vi "PID.vi"(9 "setpoint":dbl[](array[numeric])=[0.0] caption="设定值" format="%.2f", 10 "Relay":bool, 11 "Custom FPGA Reference Out":refnum<k20>) -> ()   [LabVIEW 2017, in "年前程序.lvlib"]
uses:
  <vilib>/Utility/error.llb/Error Cluster From Error Code.vi
  <vilib>/rvi/errors/niLvFpgaAdjustHostInterfaceError.vi
  <vilib>/addons/control/pid/pid.llb/PID (DBL Array).vi
  <vilib>/rvi/interface/nirviReadWriteControl/nirviReadWriteControl.xnode
  <vilib>/addons/control/pid/NI_PID_pid.lvlib
  NiFpgaLv.dll
  <vilib>/rvi/interface/Simulation/niFpgaSimulationCallBeginRW.vi
panel:
  in  "PID gains":T1={"proportional gain (Kc)"=0.0001, "integral time (Ti, min)"=3e-06, "derivative time (Td, min)"=0.0} {"proportional gain (Kc)" format="%.12f"; "integral time (Ti, min)" format="%.15f"; "derivative time (Td, min)" format="%_15f"}
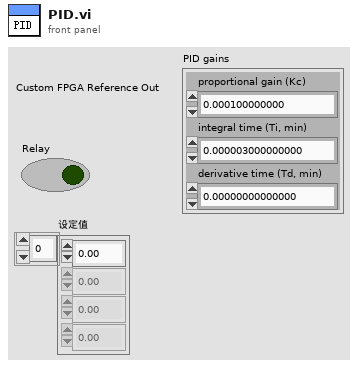
[diagram p1: front panel]
types:
  T1 = cluster{"proportional gain (Kc)":dbl, "integral time (Ti, min)":dbl, "derivative time (Td, min)":dbl}
  T2 = cluster{"proportional gain (Kc)":dbl, "integral time (Ti, min)":dbl, "derivative time (Td, min)":dbl}[]
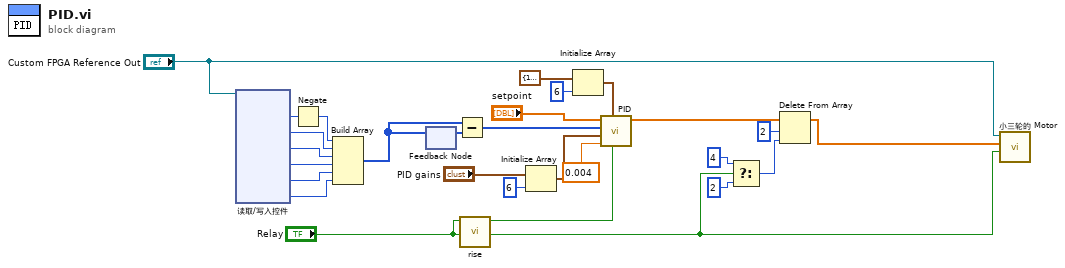
[diagram p0: block diagram]
diagram:
  n1 = xnode "读取/写入控件"("FPGA VI引用输入"="Custom FPGA Reference Out") -> ("ENC 6"=w17:i32, "ENC 1"=w18:i32, "ENC 2"=w19:i32, "ENC 3"=w13:i32, "ENC 4"=w12:i32, "ENC 5"=w11:i32)  [unwired: 1 in, 2 out]
  n2 = Negate(x=w17) -> (-x=w1:i32)
  n3 = Build Array(w1, w18, w19, w13, w12, w11) -> (w26:i32[])
  n4 = feedback #1() -> (w27:i32[])  [unwired: 1 in]
  n5 = feedback-in #1(w26) -> ()
  n6 = Subtract(x=w26, y=w27) -> (x-y=w25:i32[])
  n7 = call "rise.vi"("Signal"="Relay") -> ("Count?"=w10:bool)  [unwired: 10 in]
  n8 = Initialize Array("PID gains", 6 ("维数大小")) -> (w22:T2)
  n9 = Initialize Array(cluster{"output high":dbl, "output low":dbl} {"output high"=1.0, "output low"=-1.0} ("output range"), 6 ("维数大小")) -> (w15:cluster{"output high":dbl, "output low":dbl}[])
  n10 = call-poly <vilib>:"PID.vi"("reinitialize? (F)"=w10, "output range"=w15, "dt (s)"=0.004, "PID gains"=w22, "process variable"=w25, "setpoint"="setpoint") -> ("output"=w8:dbl[])  [unwired: 4 in, 1 out]
  n11 = Select(t=4 ("长度"), s="Relay", f=2 ("长度")) -> (s? t:f=w3:i32)
  n12 = Delete From Array(array=w8, length=2 ("长度"), index=w3) -> (array with subset deleted=w2:dbl[])  [unwired: 1 out]
  n13 = call "小三轮的 Motor.vi"("Relay"="Relay", "PWM"=w2, "Custom FPGA Reference Out"="Custom FPGA Reference Out") -> ()  [unwired: 9 in]
